vi "Calculate measured error.vi"(10 "> Cal Channel Value >":dbl[](array[numeric]), 11 "Last Cal Channel Voltage Outputted":dbl[](array[numeric])) -> (2 "Error":dbl[](array[numeric]), 3 "Measured-Desired":dbl[](array[numeric]))   [LabVIEW 2011, in "Simulated Thermocouple Custom Device.lvlib"]
uses:
  Simulated Thermocouple Custom Device.lvlib
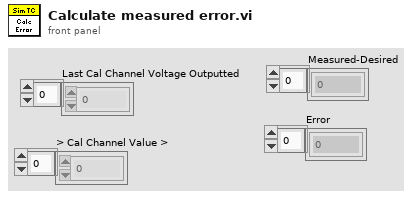
[diagram p1: front panel]
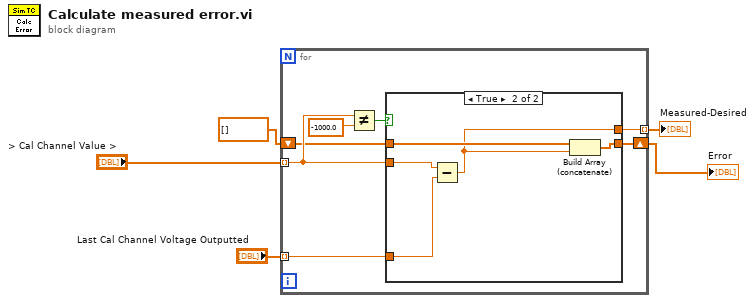
[diagram p0: block diagram]
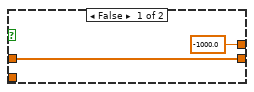
[diagram p2: hidden frame]
diagram:
  n1 = for {
    tunnel: "Last Cal Channel Voltage Outputted" -> [w12] mode=indexing
    tunnel: [w11] -> w4 mode=indexing
    tunnel: "> Cal Channel Value >" -> [w10] mode=indexing
    shift-right: [w7] -> w1
    shift-left: dbl[] [] -> [w6]
    n2 = Not Equal?(x=w10, y=-1000.0) -> (x != y?=w8:bool)
    n3 = case shown="True" w8 {
      tunnel: w12 -> [_ w16]
      tunnel: [-1000.0 w15] -> w11
      tunnel: w10 -> [_ w17]
      tunnel: [w13 w18] -> w7
      tunnel: w6 -> [w13 w19]
      frame False {
      }
      frame True {
        n4 = Subtract(x=w17, y=w16) -> (x-y=w15:dbl)
        n5 = Build Array (concatenate)(w19, w15) -> (w18:dbl[])
      }
    }
  }
  "Error" <- w1
  "Measured-Desired" <- w4
